vi "vscan.vi"(0 "IP adress":string="192.109.209.229", 1 "stop":bool, 2 "Channel":u8(ring) items=["1", "2", "3", "4", "5", "6", "7", "8", "9", "10", "11", "12", "13", "14", "15", "16"], 3 "VSCAN Parameters":T1={"tb"=5e-05, "vs_initial "=TRUE, "Voltage_step"=0.0, "Scans"=[{" vs_initial "=FALSE, "Voltage_step"=0.1, "Scan_Rate"=0.1}, {" vs_initial "=FALSE, "Voltage_step"=-0.2, "Scan_Rate"=0.1}, {" vs_initial "=FALSE, "Voltage_step"=0.0, "Scan_Rate"=0.1}], "Scan_number"=2, "N_Cycles"=0, "Record_every_dE"=0.01, "Begin_measuring_I"=0.5, "End_measuring_I"=0.75, "I_Range"=12, "E_Range"=3, "Bandwidth"=5, "em"=1, "ce"=0} {"tb" min=5e-05 max=1 format="%^_3e"; "ce" items=["Standard", "CE to ground"]; "End_measuring_I" min=0 max=1 format="%.2f"; "Begin_measuring_I" min=0 max=1 format="%.2f"; "Voltage_step" min=-10 max=10 format="%^_3e"; "N_Cycles" min=0 max=1000000; "Scan_number" min=0 max=98; "Scans"."Scan_Rate" min=1e-05 max=10 format="%^_3e"; "Scans"."Voltage_step" format="%^_3e"; "E_Range" items=["±2.5V", "±5V", "±10V", "Auto"]; "Bandwidth" items=["1"=1, "2"=2, "3"=3, "4"=4, "5"=5, "6"=6, "7"=7, "8"=8, "9"=9]; "Record_every_dE" format="%^_3e"; "I_Range" items=["1pA", "1nA", "10nA", "100nA", "1µA", "10µA", "100µA", "1mA", "10mA", "100mA", "1A", "Booster", "Auto"]}, 4 "Exit":bool, 5 "Start":bool, 6 "Draw":enum16{"I(Ewe)", "Ewe(t)", "I(t)"}(ring)=enum."Ewe(t)") -> (7 "XY Graph":cluster{"Data 101":sgl[], "Data 101":sgl[]}(graph)={"Data 101"=[8e-05, 0.1006, 0.20111999, 0.30164, 0.40219998, 0.50272, 0.60324, 0.70375997, 0.80428, 0.90484, 1.002, 1.10252, 1.20304, 1.30356, 1.40412, 1.50464, 1.60516, 1.70568, 1.8061999, 1.90676, 2.0072799, 2.1078, 2.20832, 2.3088799, 2.4094, 2.50992, 2.61044, 2.711, 2.8115199, 2.91204, 3.01256, 3.1131198, 3.21364, 3.3141599, 3.41468, 3.5152, 3.6157598, 3.71628, 3.8167999, 3.91732, 4.00108, 4.1015997, 4.20212, 4.30264, 4.4031997, 4.50372, 4.60424, 4.70476, 4.8052797, 4.90584, 5.00636, 5.1068797, 5.2074, 5.30796, 5.4084797, 5.509, 5.60952, 5.7100797, 5.8106, 5.91112], "Data 101"=[4.2835555e-07, 2.1494968e-06, 4.146294e-06, 6.138965e-06, 8.133681e-06, 1.0123058e-05, 1.2087297e-05, 1.4083101e-05, 1.6065378e-05, 1.80591e-05, 1.9984154e-05, 1.7937375e-05, 1.595267e-05, 1.3964497e-05, 1.197563e-05, 9.982255e-06, 7.9902675e-06, 6.0027883e-06, 3.9787647e-06, 1.9855738e-06, -3.2822256e-09, -1.9828094e-06, -3.9722895e-06, -5.9632257e-06, -7.95541e-06, -9.9489125e-06, -1.1902557e-05, -1.389385e-05, -1.5878555e-05, -1.7874703e-05, -1.9867039e-05, -2.1852784e-05, -2.3842693e-05, -2.583641e-05, -2.7823196e-05, -2.9813451e-05, -3.180405e-05, -3.3791526e-05, -3.5780395e-05, -3.777169e-05, -3.9435956e-05, -3.7391255e-05, -3.539476e-05, -3.3405893e-05, -3.1415642e-05, -2.9424347e-05, -2.7433402e-05, -2.5453895e-05, -2.3455323e-05, -2.1465068e-05, -1.9473428e-05, -1.7484906e-05, -1.5494306e-05, -1.3505094e-05, -1.1516228e-05, -9.523894e-06, -7.5357216e-06, -5.542347e-06, -3.5301439e-06, -1.543508e-06]}, 8 "Number of points":i32=60)   [LabVIEW 2016]
doc: "The VSCAN ( Potentiodynamic Technique) consists of scanning linearly the potential of a stationary working electrode with different scan rates.\nIn general, in this VI, the first thing to do is to start by establishing the connection with the instrument defined by its IP adress, then load the firmware in the channel selected, get the information on the plugged channels, load protocol on a channel, start/stop the protocol, retreive data and draw the graph."
uses:
  LLB/dll_Functions.llb/VSCANParameters.ctl
panel:
  in  "Display Parameters?":bool caption="Display Parameters"
  out "DllPath":path caption="DLL Path"
  out "LibVersion":string caption="DLL Version"
  out "Device Code":i32=12
  out "Exit 2":bool=TRUE
  out "Data 124":sgl[][](array[numeric])=[[8e-05, -0.00015008324, 4.2835555e-07, 0.0013634439, 1.0], [0.1006, 0.009902848, 2.1494968e-06, 0.010471455, 1.0], [0.20111999, 0.019955778, 4.146294e-06, 0.02059764, 1.0], [0.30164, 0.030008709, 6.138965e-06, 0.030609425, 1.0], [0.40219998, 0.04006164, 8.133681e-06, 0.04071481, 1.0], [0.50272, 0.050114572, 1.0123058e-05, 0.05077513, 1.0], [0.60324, 0.060167503, 1.2087297e-05, 0.06075918, 1.0], [0.70375997, 0.07022043, 1.4083101e-05, 0.07082297, 1.0], [0.80428, 0.08027337, 1.6065378e-05, 0.080852084, 1.0], [0.90484, 0.090326294, 1.80591e-05, 0.090902, 1.0], [1.002, 0.10004413, 1.9984154e-05, 0.100629516, 1.0], [1.10252, 0.0899912, 1.7937375e-05, 0.09124173, 1.0], [1.20304, 0.07993827, 1.595267e-05, 0.08120915, 1.0], [1.30356, 0.069885336, 1.3964497e-05, 0.0711627, 1.0], [1.40412, 0.059832405, 1.197563e-05, 0.06106771, 1.0], [1.50464, 0.049779475, 9.982255e-06, 0.051007397, 1.0], [1.60516, 0.039726544, 7.9902675e-06, 0.040967878, 1.0], [1.70568, 0.029673612, 6.0027883e-06, 0.030924892, 1.0], [1.8061999, 0.019620681, 3.9787647e-06, 0.020868042, 1.0], [1.90676, 0.009567751, 1.9855738e-06, 0.010804256, 1.0], [2.0072799, -0.00048518094, -3.2822256e-09, 0.0006746042, 1.0], [2.1078, -0.010538111, -1.9828094e-06, -0.009257445, 1.0], [2.20832, -0.020591041, -3.9722895e-06, -0.019307364, 1.0], [2.3088799, -0.030643972, -5.9632257e-06, -0.029412746, 1.0], [2.4094, -0.0406969, -7.95541e-06, -0.039452266, 1.0], [2.50992, -0.050749835, -9.9489125e-06, -0.049533386, 1.0], [2.61044, -0.060802765, -1.1902557e-05, -0.059479296, 1.0], [2.711, -0.07085569, -1.389385e-05, -0.06955695, 1.0], [2.8115199, -0.08090863, -1.5878555e-05, -0.07963461, 1.0], [2.91204, -0.09096155, -1.7874703e-05, -0.08969492, 1.0], [3.01256, -0.10101449, -1.9867039e-05, -0.09973444, 1.0], [3.1131198, -0.111067414, -2.1852784e-05, -0.1098225, 1.0], [3.21364, -0.12112035, -2.3842693e-05, -0.119851604, 1.0], [3.3141599, -0.13117327, -2.583641e-05, -0.12988071, 1.0], [3.41468, -0.1412262, -2.7823196e-05, -0.13995838, 1.0], [3.5152, -0.15127914, -2.9813451e-05, -0.15000136, 1.0], [3.6157598, -0.16133207, -3.180405e-05, -0.16006514, 1.0], [3.71628, -0.17138499, -3.3791526e-05, -0.1701324, 1.0], [3.8167999, -0.18143792, -3.5780395e-05, -0.18019964, 1.0], [3.91732, -0.19149086, -3.777169e-05, -0.19023915, 1.0], [4.00108, -0.1998683, -3.9435956e-05, -0.19861813, 1.0], [4.1015997, -0.18981537, -3.7391255e-05, -0.1892373, 1.0], [4.20212, -0.17976244, -3.539476e-05, -0.17914924, 1.0], [4.30264, -0.1697095, -3.3405893e-05, -0.16911319, 1.0], [4.4031997, -0.15965658, -3.1415642e-05, -0.15908061, 1.0], [4.50372, -0.14960365, -2.9424347e-05, -0.14899254, 1.0], [4.60424, -0.13955072, -2.7433402e-05, -0.13895303, 1.0], [4.70476, -0.12949778, -2.5453895e-05, -0.12891698, 1.0], [4.8052797, -0.119444855, -2.3455323e-05, -0.11883587, 1.0], [4.90584, -0.10939193, -2.1465068e-05, -0.10876862, 1.0], [5.00636, -0.09933899, -1.9473428e-05, -0.098690964, 1.0], [5.1068797, -0.08928607, -1.7484906e-05, -0.088686116, 1.0], [5.2074, -0.07923313, -1.5494306e-05, -0.07859806, 1.0], [5.30796, -0.069180205, -1.3505094e-05, -0.06854121, 1.0], [5.4084797, -0.059127275, -1.1516228e-05, -0.05848783, 1.0], [5.509, -0.049074344, -9.523894e-06, -0.048455246, 1.0], [5.60952, -0.039021414, -7.5357216e-06, -0.038367193, 1.0], [5.7100797, -0.028968483, -5.542347e-06, -0.028327677, 1.0], [5.8106, -0.018915553, -3.5301439e-06, -0.018236158, 1.0], [5.91112, -0.008862623, -1.543508e-06, -0.008182773, 1.0]] format="%.2f"
  # "Instructions:\nBefore running the VI you must type a valid IP adress that corresponds to the instrument.Then press the Run button to execute this VI.\nWhile this VI is running, choose the available channel, enter the VSCAN parameters or keep the default values, then press the button start to begin the experience.\nChoose the waveform to draw (Ewe(t) or I(t) or I(Ewe) or Ec(t). You can stop the measure if you press the stop button and exit the execution if you press the exit button."
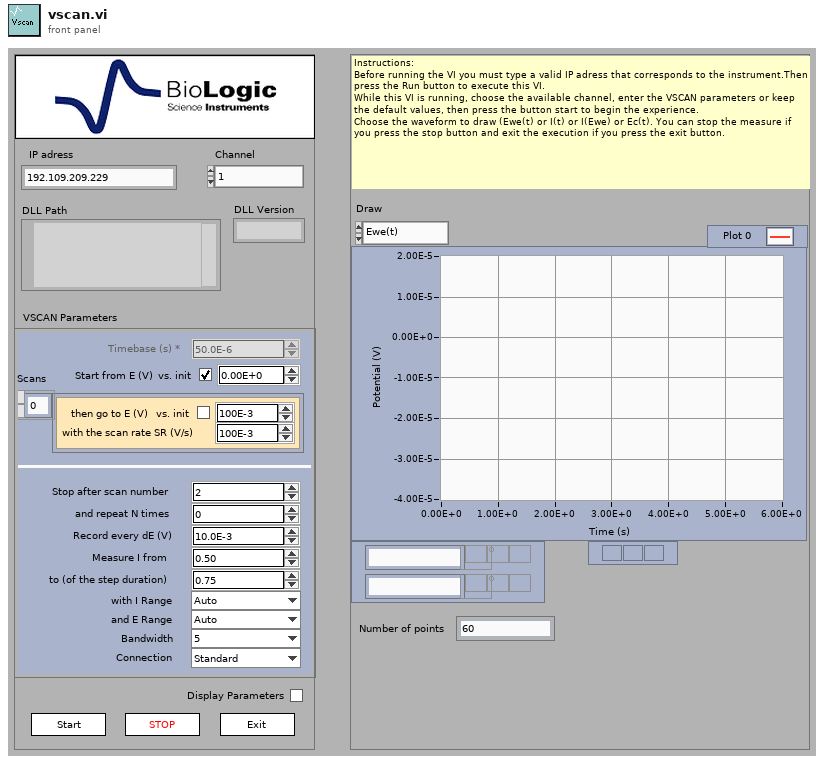
[diagram p1: front panel]
types:
  T1 = typedef "VSCANParameters.ctl" = cluster{"tb":sgl, "vs_initial ":bool, "Voltage_step":sgl, "Scans":cluster{" vs_initial ":bool, "Voltage_step":sgl, "Scan_Rate":sgl}[], "Scan_number":i32, "N_Cycles":i32, "Record_every_dE":sgl, "Begin_measuring_I":sgl, "End_measuring_I":sgl, "I_Range":u16, "E_Range":u16, "Bandwidth":u16, "em":u16, "ce":u16}
  T2 = cluster{"LibVersion":string, "StringLength":u32, "DllPath":path}
  T3 = cluster{"Channel":i32, "BoardVersion":i32, "BoardSerialCode":i32, "FirmwareCode":i32, "FirmwareVersion":i32, "XilinxVersion":i32, "AmpCode":i32, "NbAmp":i32, "LcBoard":i32, "Zboard":i32, "MuxBoard":i32, "GPRAboard":i32, "MemSize":i32, "MemFilled":i32, "state":i32, "MaxIRange":i32, "MinIRange":i32, "MaxBandwidth":i32, "NbOfTechniques":i32}
  T4 = typedef "TechniqueParameters.ctl" = cluster{"String Label":string, "Type":i32, "Valeur":i32, "Index":i32}
  T5 = cluster{"string before end tag":string, i32, i32, i32}[]
  T6 = cluster{"IRQskipped":i32, "NbRaws":i32, "NbCols":i32, "Technique Index":i32, "TechniqueID":i32, "PrcessIndex":i32, "loop":i32, "StartTime":dbl, "MuxPad":i32}
  T7 = cluster{"State":i32, "MemFilled":i32, "TimeBase":sgl, " Ewe":sgl, " EweRangeMin":sgl, " EweRangeMax":sgl, "Ece":sgl, "EceRangeMin":sgl, "EceRangeMax":sgl, "Eoverflow":i32, "I":sgl, "IRange":i32, "Ioverflow":i32, "ElapsedTime":sgl, "Freq":sgl, "Rcomp":sgl, "Saturation":sgl, "OptErr":i32, "OptPos":i32}
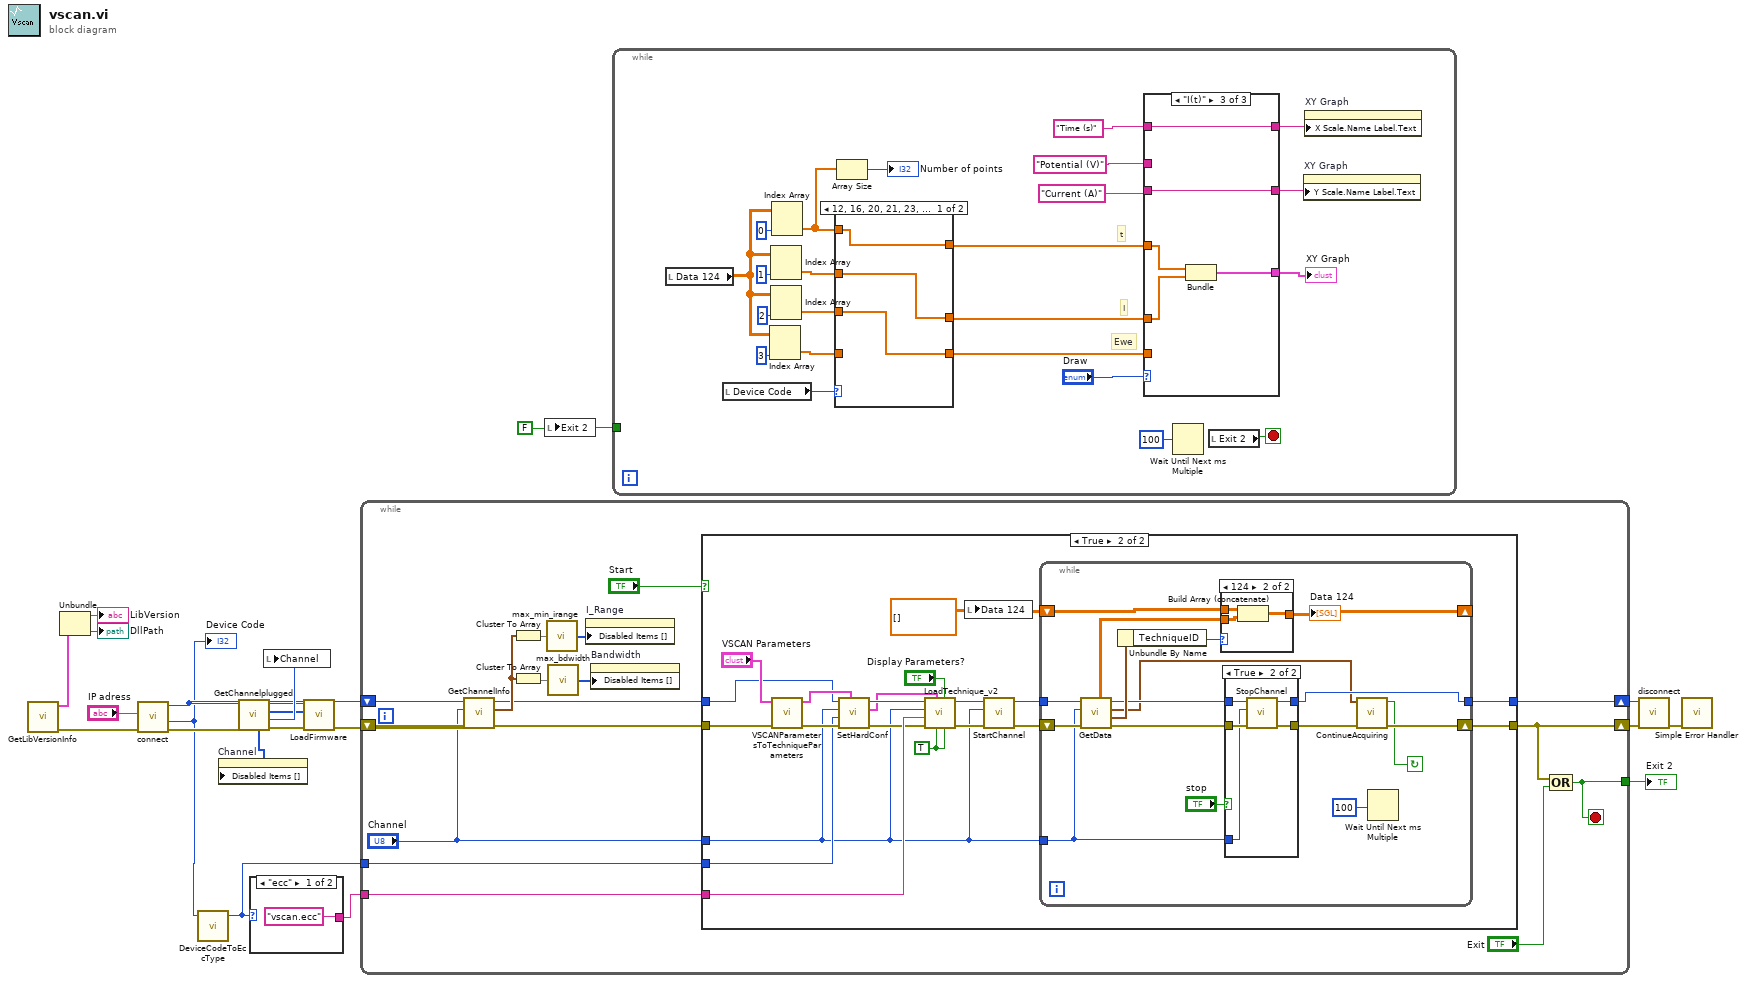
[diagram p0: block diagram]
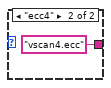
[diagram p2: hidden frame]
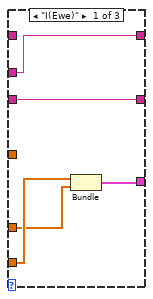
[diagram p3: hidden frame]
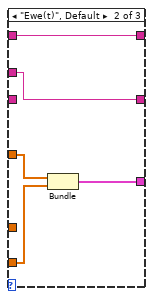
[diagram p4: hidden frame]
diagram:
  w19 = FALSE ("Exit 2")
  n1 = call "GetLibVersionInfo.vi"() -> ("error out"=w1:errorcluster, "LibInfo"=w4:T2)  [unwired: 10 in]
  n2 = Unbundle(w4) -> ("LibVersion"=→"LibVersion":string, "DllPath"=→"DllPath":path)  [unwired: 1 out]
  n3 = call "connect.vi"("error in (no error)"=w1, "IP"="IP adress") -> ("error out"=w14:errorcluster, "Device Code"=w8:i32, "ID Out"=w16:i32)  [unwired: 6 in, 1 out]
  "Device Code" <- w8
  n4 = call "DeviceCodeToEccType.vi"("Device Code"=w8) -> ("EccType"=w5:enum16{"ecc", "ecc4"})  [unwired: 4 in]
  n5 = call "GetChannelplugged.vi"("error in (no error)"=w14, "ID In"=w16) -> ("error out"=w13:errorcluster, "FirstPluggedChannel"=w17:u8, "PluggedChannels"=w11:u8[], "DisabledChannels"=w12:i32[])  [unwired: 5 in, 1 out]
  n6 = property on="Channel" class="Ring (strict)"("Disabled Items []"=w12) -> ()  [unwired: 2 in, 2 out]
  n7 = case shown="\"ecc\"" w5 {
    tunnel: ["vscan.ecc" ("FName") "vscan4.ecc" ("FName")] -> w7
    frame "ecc" {
    }
    frame "ecc4" {
    }
  }
  n8 = local write "Channel"(w17) -> ()
  n9 = call "LoadFirmware.vi"("error in (no error)"=w13, "Channels"=w11, "ID In"=w16) -> ("error out"=w10:errorcluster)  [unwired: 6 in, 2 out]
  n10 = while {
    shift-right: [w25] -> w9
    shift-left: w10 -> [w32]
    tunnel: [w23] -> w20
    tunnel: w5 -> [w33]
    shift-right: [w26] -> w15
    shift-left: w16 -> [w34]
    tunnel: w7 -> [w27]
    stop <- w23 stop-if-true
    n11 = call "GetChannelInfo.vi"("error in (no error)"=w32, "Channel"="Channel", "ID"=w34) -> ("error out"=w31:errorcluster, "Channel information"=w29:T3, "ID Out"=w28:i32)  [unwired: 6 in]
    n12 = Cluster To Array(cluster=w29) -> (array=w38:i32[])
    n13 = Cluster To Array(cluster=w29) -> (array=w37:i32[])
    n14 = call "max_min_irange.vi"("resources"=w38) -> ("disabled ranges"=w35:i32[])
    n15 = call "max_bdwidth.vi"("resources"=w37) -> ("disabled ranges"=w36:i32[])
    n16 = property on="I_Range" class="Ring (strict)"("Disabled Items []"=w35) -> ()  [unwired: 2 in, 2 out]
    n17 = property on="Bandwidth" class="Ring (strict)"("Disabled Items []"=w36) -> ()  [unwired: 2 in, 2 out]
    n18 = case shown="True" "Start" {
      tunnel: "Channel" -> [_ w43]
      tunnel: [w41 w52] -> w25
      tunnel: w31 -> [w41 w60]
      tunnel: w33 -> [_ w44]
      tunnel: w28 -> [w40 w45]
      tunnel: w27 -> [_ w57]
      tunnel: [w40 w51] -> w26
      frame False {
      }
      frame True {
        w58 = TRUE ("First Protocol")
        w61 = sgl[][] []
        n19 = call "VSCANParametersToTechniqueParameters.vi"("error in (no error)"=w60, "VSCAN Parameters"="VSCAN Parameters") -> ("error out"=w50:errorcluster, "TechniquesParameters"=w46:T4[])  [unwired: 8 in]
        n20 = call "SetHardConf.vi"("Params Values"=w46, "error in (no error)"=w50, "EccType"=w44, "Channel"=w43, "ID In"=w45) -> ("error out"=w49:errorcluster, "Params Values Trimed"=w47:T5, "ID Out"=w48:i32)  [unwired: 4 in]
        n21 = call "LoadTechnique_v2.vi"("Last Protocol"=w58, "Display Parameters?"="Display Parameters?", "First Protocol"=w58, "TechniqueParameters"=w47, "error in (no error)"=w49, "FName"=w57, "Selected Channel"=w43, "ID In"=w48) -> ("error out"=w56:errorcluster, "ID  Out"=w55:i32)  [unwired: 2 in]
        n22 = local write "Data 124"(w61) -> ()
        n23 = call "StartChannel.vi"("error in (no error)"=w56, "Channel"=w43, "ID In"=w55) -> ("error out"=w54:errorcluster, "ID Out"=w53:i32)  [unwired: 7 in]
        n24 = while {
          shift-right: [w65] -> w52
          shift-left: w54 -> [w77]
          shift-right: [w74] -> _
          shift-left: w61 -> [w75]
          tunnel: w43 -> [w67]
          tunnel: w53 -> [w69]
          tunnel: [w66] -> w51
          stop <- w63 continue-if-true
          n25 = call "GetData.vi"("error in (no error)"=w77, "Channel"=w67, "ID In"=w69) -> ("error out"=w73:errorcluster, "Data information"=w78:T6, "Current values"=w62:T7, "ID Out"=w68:i32, "Data"=w70:dbl[][])  [unwired: 4 in]
          n26 = Unbundle By Name(w78) -> ("TechniqueID"=w72:i32)
          n27 = case shown="124" w72 {
            tunnel: w70 -> [_ w89]
            tunnel: w75 -> [w86 w88]
            tunnel: [w86 w87] -> w74
            frame 0, Default {
            }
            frame 124 {
              n28 = Build Array (concatenate)(w88, w89) -> (w87:dbl[][])
            }
          }
          "Data 124" <- w74
          n29 = case shown="True" "stop" {
            tunnel: [w80 w85] -> w64
            tunnel: w73 -> [w80 w84]
            tunnel: w68 -> [w79 w83]
            tunnel: w67 -> [_ w82]
            tunnel: [w79 w81] -> w66
            frame False {
            }
            frame True {
              n30 = call "StopChannel.vi"("error in (no error)"=w84, "Channel"=w82, "ID In"=w83) -> ("error out"=w85:errorcluster, "ID Out"=w81:i32)  [unwired: 7 in]
            }
          }
          n31 = call "ContinueAcquiring.vi"("error in"=w64, "Current values"=w62) -> ("error out"=w65:errorcluster, "ContinueAcquiring?"=w63:bool)  [unwired: 8 in]
          n32 = Wait Until Next ms Multiple(millisecond multiple=u32 100) -> ()  [unwired: 1 out]
        }
      }
    }
    n33 = Compound Arithmetic op=OR(w25, "Exit") -> (w23:bool)
  }
  "Exit 2" <- w20
  n34 = local write "Exit 2"(w19) -> ()
  n35 = while {
    tunnel: w19 -> [_]
    stop <- w111 stop-if-true
    # "Ewe"
    # "I"
    # "t"
    n36 = local read "Data 124"() -> (w102:sgl[][])
    n37 = local read "Device Code"() -> (w100:i32)
    n38 = Index Array(array=w102, index (col)=3 ("Index")) -> (element=w104:sgl[])  [unwired: 1 in]
    n39 = Index Array(array=w102, index (col)=1 ("Index")) -> (element=w107:sgl[])  [unwired: 1 in]
    n40 = Index Array(array=w102, index (col)=2 ("Index")) -> (element=w105:sgl[])  [unwired: 1 in]
    n41 = Index Array(array=w102, index (col)=0 ("Index")) -> (element=w101:sgl[])  [unwired: 1 in]
    n42 = case shown="12, 16, 20, 21, 23, 27" w100 {
      tunnel: w107 -> [w129 _]
      tunnel: w105 -> [w128 w132]
      tunnel: w104 -> [_ w131]
      tunnel: w101 -> [w130 w133]
      tunnel: [w130 w133] -> w92
      tunnel: [w129 w132] -> w91
      tunnel: [w128 w131] -> w90
      frame 12, 16, 20, 21, 23, 27 {
      }
      frame Default {
      }
    }
    n43 = Array Size(array=w101) -> (size(s)=→"Number of points":i32)
    n44 = case shown="\"I(t)\"" "Draw" {
      tunnel: w92 -> [_ w122 w127]
      tunnel: w91 -> [w114 _ w126]
      tunnel: [w113 w118 w123] -> w99
      tunnel: "Potential (V)" ("Y Scale.Name Label.Text") -> [w117 w121 _]
      tunnel: "Current (A)" ("Y Scale.Name Label.Text") -> [w116 _ w125]
      tunnel: [w116 w121 w125] -> w97
      tunnel: [w117 w120 w124] -> w96
      tunnel: "Time (s)" ("Y Scale.Name Label.Text") -> [_ w120 w124]
      tunnel: w90 -> [w115 w119 _]
      frame "I(Ewe)" {
        n45 = Bundle("Data 124"=w115, "Data 124"=w114) -> (w113:cluster{"Data 124":sgl[], "Data 124":sgl[]})  [unwired: 1 in]
      }
      frame "Ewe(t)", Default {
        n46 = Bundle("Data 124"=w122, "Data 124"=w119) -> (w118:cluster{"Data 124":sgl[], "Data 124":sgl[]})  [unwired: 1 in]
      }
      frame "I(t)" {
        n47 = Bundle("Data 124"=w127, "Data 124"=w126) -> (w123:cluster{"Data 124":sgl[], "Data 124":sgl[]})  [unwired: 1 in]
      }
    }
    "XY Graph" <- w99
    n48 = Wait Until Next ms Multiple(millisecond multiple=u32 100) -> ()  [unwired: 1 out]
    n49 = local read "Exit 2"() -> (w111:bool)
    n50 = property on="XY Graph" class="XYGraph (strict)"("Y Scale.Name Label.Text"=w97) -> ()  [unwired: 2 in, 2 out]
    n51 = property on="XY Graph" class="XYGraph (strict)"("X Scale.Name Label.Text"=w96) -> ()  [unwired: 2 in, 2 out]
  }
  n52 = call "disconnect.vi"("error in (no error)"=w9, "ID In"=w15) -> ("error out"=w6:errorcluster)  [unwired: 9 in]
  n53 = call <vilib>:"Simple Error Handler.vi"("error in (no error)"=w6) -> ()  [unwired: 4 in, 5 out]
